vi "RT Animation.vi"(0 "3D Picture":refnum<vi>, 2 "RT Position":T3, 3 "Left/Right":bool=TRUE, 4 "Arm Refs":T1) -> ()   [LabVIEW 2010]
uses:
  <vilib>/Analysis/Matrix/Datatypes/RealMatrix.ctl
  <vilib>/picture/3D Picture Control/NI_3D Picture Control.lvlib
  <vilib>/Analysis/Matrix/NI_Matrix.lvlib
panel:
  # "Left"
  # "Right"
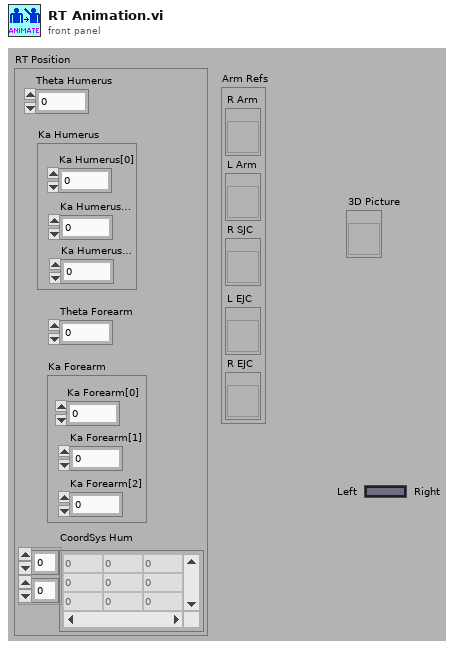
[diagram p1: front panel]
types:
  T1 = cluster{"R Arm":refnum<vi>, "L Arm":refnum<vi>, "R SJC":refnum<vi>, "L EJC":refnum<vi>, "R EJC":refnum<vi>}
  T2 = typedef "NI_Matrix.lvlib/RealMatrix.ctl" = dbl[][]
  T3 = cluster{"Theta Humerus":dbl, "Ka Humerus":cluster{"Ka Humerus[0]":dbl, "Ka Humerus[1]":dbl, "Ka Humerus[2]":dbl}, "Theta Forearm":dbl, "Ka Forearm":cluster{"Ka Forearm[0]":dbl, "Ka Forearm[1]":dbl, "Ka Forearm[2]":dbl}, "CoordSys Hum":T2}
  T4 = cluster{"Ka Humerus[0]":dbl, "Ka Humerus[1]":dbl, "Ka Humerus[2]":dbl}
  T5 = cluster{"Ka Forearm[0]":dbl, "Ka Forearm[1]":dbl, "Ka Forearm[2]":dbl}
  T6 = cluster{dbl, "Ka Humerus[0]":dbl, "Ka Humerus[0]":dbl}
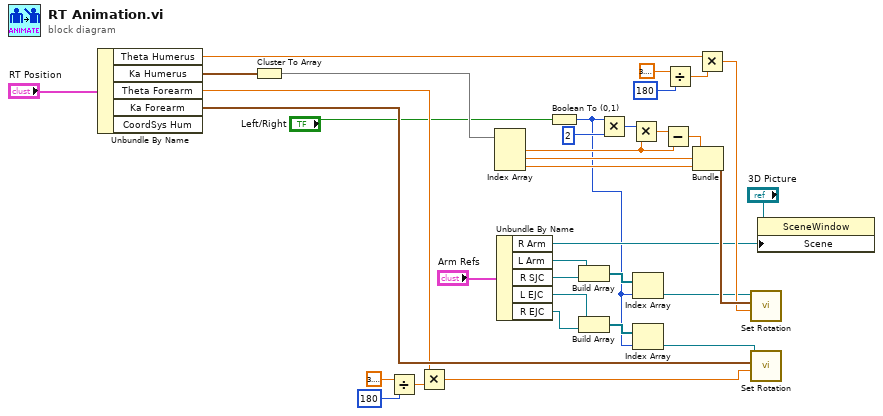
[diagram p0: block diagram]
diagram:
  n1 = Unbundle By Name("RT Position") -> ("Theta Humerus"=w17:dbl, "Ka Humerus"=w30:T4, "Theta Forearm"=w10:dbl, "Ka Forearm"=w35:T5)  [unwired: 1 out]
  n2 = Cluster To Array(cluster=w30) -> (array=w4:dbl[])
  n3 = Divide(x=3.141592653589793, y=180) -> (x/y=w13:dbl)
  n4 = Multiply(x=w10, y=w13) -> (x*y=w9:dbl)
  n5 = Index Array(array=w4) -> (element #1=w8:dbl, element #2=w28:dbl, element #3=w27:dbl)  [unwired: 3 in]
  n6 = Unbundle By Name("Arm Refs") -> ("R Arm"=w5:refnum<vi>, "L Arm"=w26:refnum<vi>, "R SJC"=w25:refnum<vi>, "L EJC"=w23:refnum<vi>, "R EJC"=w22:refnum<vi>)
  n7 = Boolean To (0,1)(Boolean="Left/Right") -> (0, 1=w1:i16)
  n8 = Build Array(w26, w25) -> (w24:refnum<vi>[])
  n9 = Build Array(w23, w22) -> (w21:refnum<vi>[])
  n10 = Multiply(x=w1, y=i16 2) -> (x*y=w32:i16)
  n11 = Multiply(x=w32, y=w8) -> (x*y=w31:dbl)
  n12 = Index Array(array=w24, index=w1) -> (element=w3:refnum<vi>)
  n13 = Index Array(array=w21, index=w1) -> (element=w14:refnum<vi>)
  n14 = Subtract(x=w31, y=w8) -> (x-y=w29:dbl)
  n15 = Divide(x=3.141592653589793, y=180) -> (x/y=w16:dbl)
  n16 = Bundle(w29, "Ka Humerus[0]"=w28, "Ka Humerus[0]"=w27) -> (w20:T6)  [unwired: 1 in]
  n17 = Multiply(x=w17, y=w16) -> (x*y=w15:dbl)
  n18 = call <vilib>:"Set Rotation.vi"("Angle"=w15, "Axis"=w20, "Scene Object"=w3) -> ()  [unwired: 7 in, 2 out]
  n19 = call <vilib>:"Set Rotation.vi"("Angle"=w9, "Axis"=w35, "Scene Object"=w14) -> ()  [unwired: 7 in, 2 out]
  n20 = property class="SceneWindow"(reference="3D Picture", "Scene"=w5) -> ()  [unwired: 1 in, 2 out]
